vi "N-664 Stage Engine.vi"(0 "Unique Notifier Name":string, 11 "COM Port":string[](array[string])) -> ()   [LabVIEW 2016]
uses:
  Stages Controls/Stage Focus Control.ctl
  Stages Controls/Stage Status.ctl
  Stages Controls/Stage Notifier Element.ctl
  Stages Controls/Stage Actions.ctl
  <vilib>/Instr/_visa.llb/VISA Configure Serial Port (Instr).vi
panel:
  in  "ReInitialize":bool
  in  "Abort":bool
  in  "Velocity":dbl(ring)=2.0 items=["SUPER SLOW"=0.0010000000474974513, "SLOW"=1.0, "MEDIUM"=2.0, "FAST"=3.0]
  out "Status":T1
  in  "QUIT":bool
  in  "Focus Control":T2
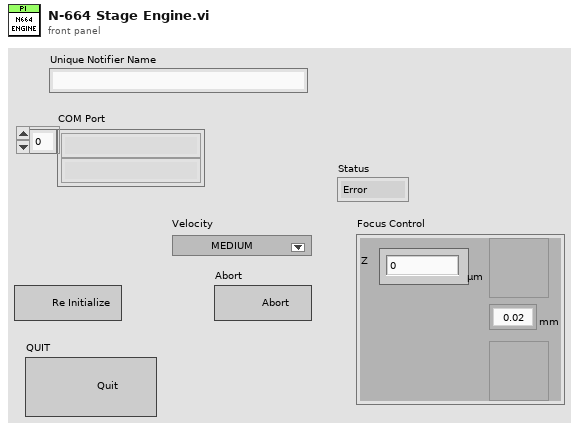
[diagram p1: front panel]
types:
  T1 = typedef "Stage Status.ctl" = enum16{"Error", "Abort", "Busy", "On Target"}
  T2 = typedef "Stage Focus Control.ctl" = cluster{"Focus Step (um)":enum16{"0.02", "0.05", "0.1", "0.5", "1", "2", "5", "10", "20"}, "Focus Up":bool, "Focus Down":bool, "Z ":dbl}
  T3 = typedef "Stage Actions.ctl" = enum16{"Get Position", "MVR", "MOVE", "HALT", "ONTARGET", "ERROR", "REFERENCE", "INIT", "VELOCITY", "STATUS", "EXIT", "HOME", "ZEROPOS", "NANOPOS", "ANALOG", "QUIT"}
  T4 = typedef "Stage Notifier Element.ctl" = cluster{"Action":T3, "Axis":bool[], "Setpoint":dbl[], "Velocity":dbl, "Cmd Recvd?":bool, "Position":dbl[], "Status":T1, "Misc":variant}
  T5 = cluster{"Focus Step (um)":bool, "Focus Up":bool, "Focus Down":bool, "Z ":bool}
  T6 = enum16{"0.02", "0.05", "0.1", "0.5", "1", "2", "5", "10", "20"}
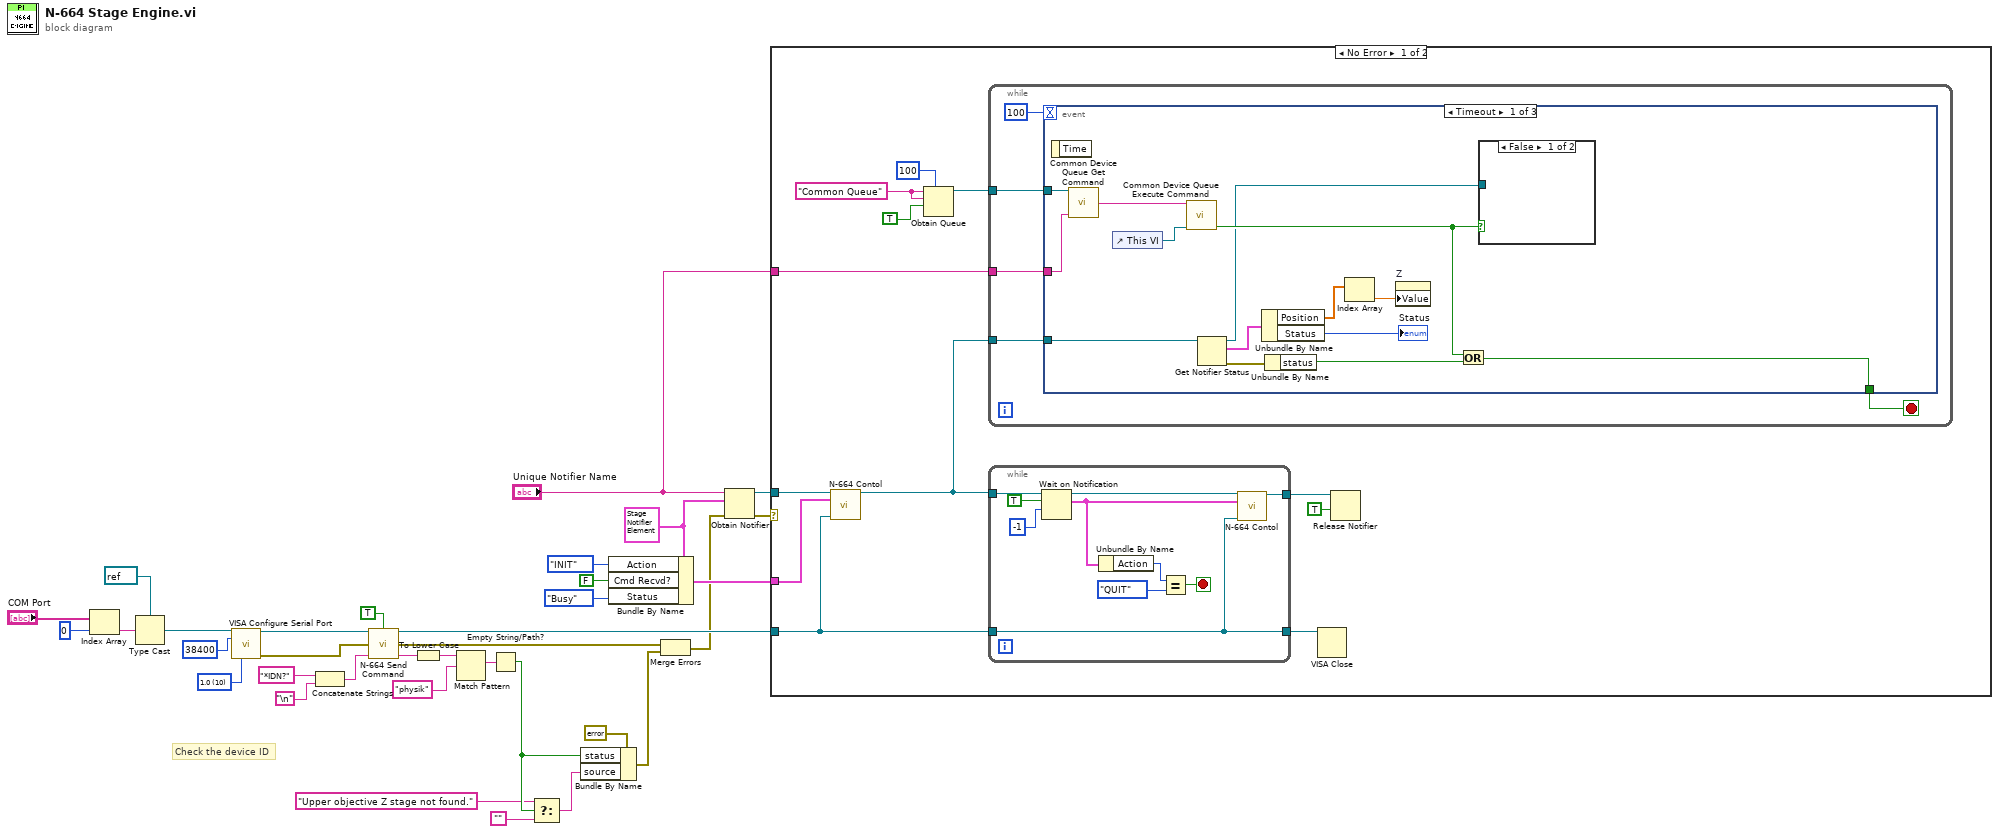
[diagram p0: block diagram]
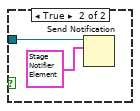
[diagram p2: hidden frame]
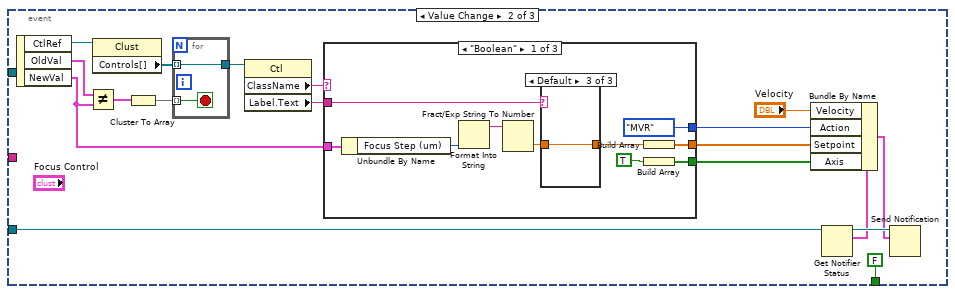
[diagram p3: hidden frame]
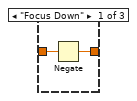
[diagram p4: hidden frame]
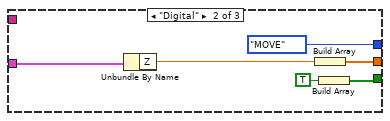
[diagram p6: hidden frame]
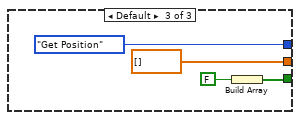
[diagram p7: hidden frame]
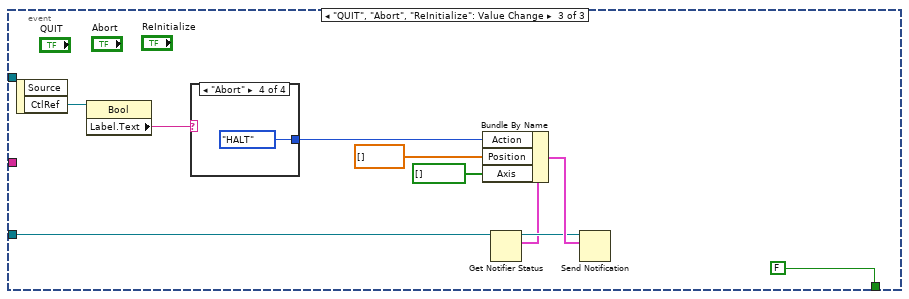
[diagram p8: hidden frame]
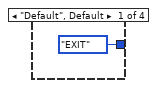
[diagram p9: hidden frame]
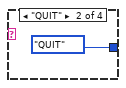
[diagram p10: hidden frame]
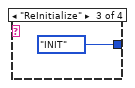
[diagram p11: hidden frame]
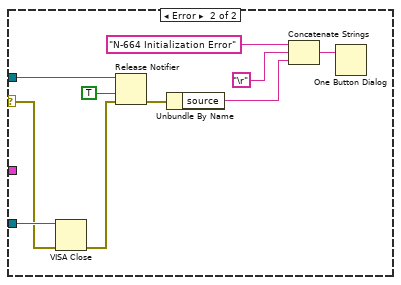
[diagram p12: hidden frame]
diagram:
  w27 = u16 10 items=["1.0"=10, "1.5"=15, "2.0"=20] ("stop bits (10: 1 bit)")
  w28 = T4 {"Action"=enum."Get Position", "Axis"=[], "Setpoint"=[], "Velocity"=0.5, "Cmd Recvd?"=FALSE, "Position"=[], "Status"=enum."Abort", "Misc"=variant} ("Stage Status")
  # "Check the device ID"
  n1 = Index Array(array="COM Port", index=0) -> (element=w33:string)
  n2 = Type Cast(type=refnum<visa-resource-name> refnum ("reference out"), x=w33) -> (*(type *) &x=w20:refnum<visa-resource-name>)
  n3 = call-poly "VISA Configure Serial Port"("VISA resource name"=w20, "baud rate (9600)"=u32 38400, "stop bits (10: 1 bit)"=w27) -> ("VISA resource name out"=w19:refnum<visa-resource-name>, "error out"=w18:errorcluster)  [unwired: 11 in]
  n4 = Concatenate Strings("*IDN?" ("string"), "\n") -> (w15:string)
  n5 = call "N-664 Send Command.vi"("VISA Ref"=w19, "Wait for Reply?"=TRUE, "Error In"=w18, "Command"=w15) -> ("VISA Ref Out"=w17:refnum<visa-resource-name>, "Error Out"=w6:errorcluster, "Response"=w8:string)  [unwired: 9 in]
  n6 = To Lower Case(string=w8) -> (all lower case string=w11:string)
  n7 = Match Pattern(string=w11, regular expression="physik" ("string")) -> (match substring=w10:string)  [unwired: 1 in, 3 out]
  n8 = Empty String/Path?(string/path=w10) -> (empty?=w4:bool)
  n9 = Select(t="Upper objective Z stage not found." ("string"), s=w4, f="") -> (s? t:f=w3:string)
  n10 = Bundle By Name(cluster=errorcluster {"status"=FALSE, "code"=0, "source"=""} ("Error Out"), "status"=w4, "source"=w3) -> (w5:errorcluster)
  n11 = Bundle By Name(cluster=w28, "Action"=Stage_Actions."INIT", "Cmd Recvd?"=FALSE, "Status"=Stage_Status."Busy") -> (w23:T4)
  n12 = Merge Errors(w6, w5) -> (w16:errorcluster)
  n13 = Obtain Notifier(name (unnamed)="Unique Notifier Name", notification data type=w28, error in (no error)=w16) -> (notifier out=w25:refnum<notifier>, error out=w24:errorcluster)  [unwired: 1 in, 1 out]
  n14 = case shown="No Error" w24 {
    selector: w24 -> [_ w136]
    tunnel: w17 -> [w41 w137]
    tunnel: w25 -> [w45 w138]
    tunnel: w23 -> [w44 _]
    tunnel: "Unique Notifier Name" -> [w35 _]
    frame No Error {
      w39 = "Common Queue" ("Unique Notifier Name")
      n15 = call "N-664 Contol.vi"("N-664 Notifier"=w45, "Stage Action"=w44, "VISA In"=w41) -> ("N-664 Notifier (Dup)"=w43:refnum<notifier>)  [unwired: 12 in]
      n16 = Obtain Queue(max queue size (-1, unlimited)=100, name (unnamed)=w39, element data type=w39, create if not found? (T)=TRUE) -> (queue out=w36:refnum<queue>)  [unwired: 1 in, 2 out]
      n17 = while {
        tunnel: w43 -> [w59]
        tunnel: w36 -> [w58]
        tunnel: w35 -> [w57]
        stop <- w60 stop-if-true
        n18 = event shown="[0] Timeout" {
          selector: _ -> [_ _ _]
          dyn-events: _ -> [_ _ _]
          timeout: 100 -> [_ _ _]
          tunnel: [w65 FALSE ("status") FALSE ("status")] -> w60
          tunnel: w59 -> [w74 w83 w127]
          tunnel: w58 -> [w67 _ _]
          tunnel: w57 -> [w62 _ _]
          event Timeout {
            n19 = event-data() -> ()  [unwired: 1 in, 1 out]
            n20 = call "Common Device Queue Get Command.vi"("Common Queue"=w67, "Notifier Name"=w62) -> ("Command"=w68:string)  [unwired: 12 in, 1 out]
            n21 = control-ref of="This VI"() -> (w69:refnum<vi>)
            n22 = call "Common Device Queue Execute Command.vi"("Common Command"=w68, "VI Refnum"=w69) -> ("Quit?"=w64:bool)  [unwired: 12 in, 1 out]
            n23 = Get Notifier Status(notifier=w74) -> (notifier out=w63:refnum<notifier>, current notification=w73:T4, error out=w71:errorcluster)  [unwired: 1 in, 2 out]
            n24 = Unbundle By Name(w73) -> ("Position"=w72:dbl[], "Status"=→"Status":T1)
            n25 = Unbundle By Name(w71) -> ("status"=w66:bool)
            n26 = Index Array(array=w72) -> (element=w75:dbl)  [unwired: 1 in]
            n27 = property on="Z" class="DigNum (strict)"("Value"=w75) -> ()  [unwired: 2 in, 2 out]
            n28 = Or(x=w64, y=w66) -> (x .or. y?=w65:bool)
            n29 = case shown="False" w64 {
              tunnel: w63 -> [_ w77]
              frame False {
              }
              frame True {
                n30 = Send Notification(notification=T4 {"Action"=enum."QUIT", "Axis"=[], "Setpoint"=[], "Velocity"=0.5, "Cmd Recvd?"=FALSE, "Position"=[], "Status"=enum."Error", "Misc"=variant} ("Stage Status"), notifier=w77) -> ()  [unwired: 1 in, 2 out]
              }
            }
          }
          event Value Change {
            n31 = event-data() -> ("CtlRef"=w94:refnum<vi>, "OldVal"=w95:T2, "NewVal"=w88:T2)  [unwired: 1 in]
            n32 = Not Equal?(x=w95, y=w88) -> (x != y?=w93:T5)
            n33 = property class="Clust"(reference=w94) -> ("Controls[]"=w91:refnum<vi>[])  [unwired: 1 in, 2 out]
            n34 = Cluster To Array(cluster=w93) -> (array=w92:bool[])
            n35 = for {
              tunnel: w92 -> [w121] mode=indexing
              tunnel: [w120] -> w90
              tunnel: w91 -> [w120] mode=indexing
              stop <- w121 stop-if-true
            }
            n36 = property class="Ctl"(reference=w90) -> ("ClassName"=w89:string, "Label.Text"=w87:string)  [unwired: 1 in, 2 out]
            n37 = case shown="\"Boolean\"" w89 {
              tunnel: w88 -> [w103 w115 _]
              tunnel: w87 -> [w104 _ _]
              tunnel: [w98 w113 dbl[] []] -> w86
              tunnel: [w97 w112 w118] -> w85
              tunnel: [Stage_Actions."MVR" ("Action") Stage_Actions."MOVE" ("Action") Stage_Actions."Get Position" ("Action")] -> w82
              frame "Boolean" {
                n38 = Unbundle By Name(w103) -> ("Focus Step (um)"=w101:T6)
                n39 = Format Into String(w101) -> (resulting string=w102:string)  [unwired: 3 in, 1 out]
                n40 = Fract/Exp String To Number(string=w102) -> (number=w100:dbl)  [unwired: 3 in, 1 out]
                n41 = case shown="Default" w104 {
                  tunnel: w100 -> [w107 w108 w109]
                  tunnel: [w106 w108 w109] -> w99
                  frame "Focus Down" {
                    n42 = Negate(x=w107) -> (-x=w106:dbl)
                  }
                  frame "Focus Up" {
                  }
                  frame Default {
                  }
                }
                n43 = Build Array(w99) -> (w98:dbl[])
                n44 = Build Array(TRUE) -> (w97:bool[])
              }
              frame "Digital" {
                n45 = Unbundle By Name(w115) -> ("Z"=w114:dbl)
                n46 = Build Array(w114) -> (w113:dbl[])
                n47 = Build Array(TRUE) -> (w112:bool[])
              }
              frame Default {
                n48 = Build Array(FALSE) -> (w118:bool[])
              }
            }
            n49 = Get Notifier Status(notifier=w83) -> (notifier out=w81:refnum<notifier>, current notification=w80:T4)  [unwired: 1 in, 3 out]
            n50 = Bundle By Name(cluster=w80, "Velocity"="Velocity", "Action"=w82, "Setpoint"=w86, "Axis"=w85) -> (w79:T4)
            n51 = Send Notification(notification=w79, notifier=w81) -> ()  [unwired: 1 in, 2 out]
          }
          event "QUIT", "Abort", "ReInitialize": Value Change {
            n52 = event-data() -> ("CtlRef"=w124:refnum<vi>)  [unwired: 1 in, 1 out]
            n53 = property class="Bool"(reference=w124) -> ("Label.Text"=w123:string)  [unwired: 1 in, 2 out]
            n54 = case shown="\"Abort\"" w123 {
              tunnel: [Stage_Actions."EXIT" ("Action") Stage_Actions."QUIT" ("Action") Stage_Actions."INIT" ("Action") Stage_Actions."HALT" ("Action")] -> w122
              frame "Default", Default {
              }
              frame "QUIT" {
              }
              frame "ReInitialize" {
              }
              frame "Abort" {
              }
            }
            n55 = Get Notifier Status(notifier=w127) -> (notifier out=w126:refnum<notifier>, current notification=w125:T4)  [unwired: 1 in, 3 out]
            n56 = Bundle By Name(cluster=w125, "Action"=w122, "Position"=dbl[] [], "Axis"=bool[] []) -> (w128:T4)
            n57 = Send Notification(notification=w128, notifier=w126) -> ()  [unwired: 1 in, 2 out]
          }
        }
      }
      n58 = while {
        tunnel: w43 -> [w54]
        tunnel: [w50] -> w42
        tunnel: w41 -> [w49]
        tunnel: [w49] -> w40
        stop <- w56 stop-if-true
        n59 = Wait on Notification(notifier=w54, ignore previous (F)=TRUE, timeout in ms (-1)=-1) -> (notifier out=w51:refnum<notifier>, notification=w48:T4)  [unwired: 1 in, 2 out]
        n60 = Unbundle By Name(w48) -> ("Action"=w47:T3)
        n61 = Equal?(x=w47, y=Stage_Actions."QUIT") -> (x = y?=w56:bool)
        n62 = call "N-664 Contol.vi"("N-664 Notifier"=w51, "Stage Action"=w48, "VISA In"=w49) -> ("N-664 Notifier (Dup)"=w50:refnum<notifier>)  [unwired: 12 in]
      }
      n63 = VISA Close(VISA resource name=w40) -> ()  [unwired: 1 in, 1 out]
      n64 = Release Notifier(notifier=w42, force destroy? (F)=TRUE) -> ()  [unwired: 1 in, 3 out]
    }
    frame Error {
      n65 = VISA Close(VISA resource name=w137, error in (no error)=w136) -> (error out=w139:errorcluster)
      n66 = Release Notifier(notifier=w138, force destroy? (F)=TRUE, error in (no error)=w139) -> (error out=w144:errorcluster)  [unwired: 2 out]
      n67 = Unbundle By Name(w144) -> ("source"=w141:string)
      n68 = Concatenate Strings("N-664 Initialization Error", "\r", w141) -> (w140:string)
      n69 = One Button Dialog(message=w140) -> ()  [unwired: 1 in, 1 out]
    }
  }
